vi "Formato de Archivo.vi"(8 "error in (no error)":errorcluster, 10 "Formato":enum16{"TXT", "TDMS"}(ring), 11 "Generador de Funciones in":refnum<class "Generador de Funciones.lvclass">) -> (0 "error out":errorcluster, 3 "Generador de Funciones out":refnum<class "Generador de Funciones.lvclass">)   [LabVIEW 2020, in "Generador de Funciones.lvlib" / "Generador de Funciones.lvclass"]
uses:
  Generador de Funciones.lvclass
  C:/Program Files (x86)/National Instruments/LabVIEW 2020/vi.lib/ActorFramework/Actor/Actor.lvclass
  Generador de Funciones.lvclass/Generador de Funciones.ctl
  Loggin/Loggin/Loggin.lvclass
  TDMS/TDMS/TDMS.lvclass
  <vilib>/ActorFramework/Message Enqueuer/Message Enqueuer.lvclass/Message Enqueuer.ctl
  <vilib>/ActorFramework/Message Enqueuer/Enqueue.vi
  <vilib>/ActorFramework/Stop Msg/Stop Msg.lvclass
  C:/Program Files (x86)/National Instruments/LabVIEW 2020/vi.lib/ActorFramework/Message/Message.lvclass
  <vilib>/ActorFramework/Message Priority Queue/Priority Enqueue.vi
  <vilib>/ActorFramework/Actor/Actor.lvclass
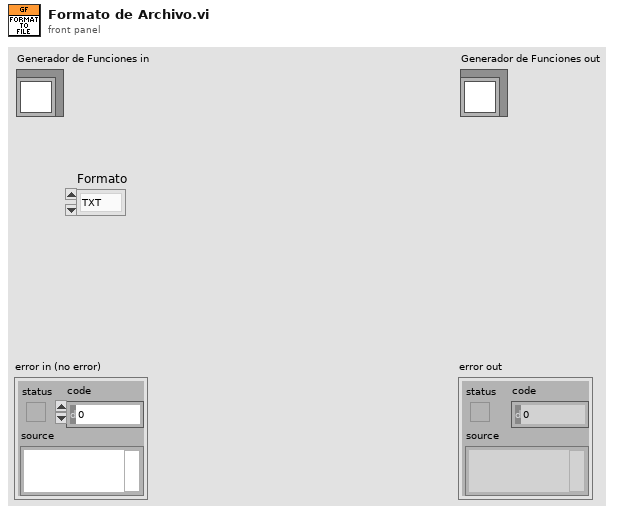
[diagram p1: front panel]
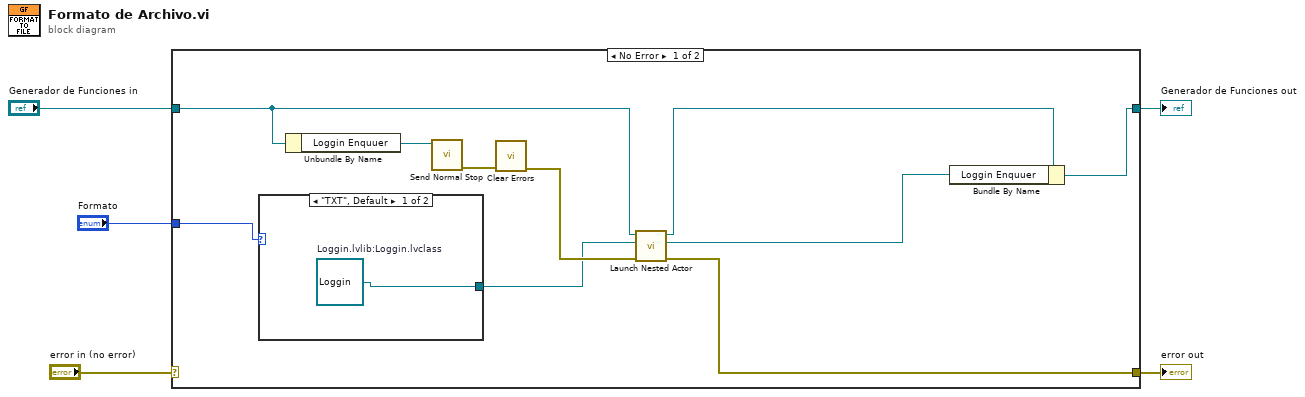
[diagram p0: block diagram]
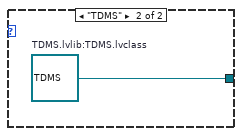
[diagram p2: hidden frame]
diagram:
  n1 = case shown="No Error" "error in (no error)" {
    selector: "error in (no error)" -> [_ w19]
    tunnel: [w10 w19] -> w4
    tunnel: [w8 w18] -> w2
    tunnel: "Generador de Funciones in" -> [w12 w18]
    tunnel: "Formato" -> [w13 _]
    frame No Error {
      n2 = case shown="\"TXT\", Default" w13 {
        tunnel: [w16 w17] -> w6
        frame "TXT", Default {
          w16 = refnum<class "Loggin.lvclass"> refnum  # Loggin.lvlib:Loggin.lvclass
        }
        frame "TDMS" {
          w17 = refnum<class "TDMS.lvclass"> refnum  # TDMS.lvlib:TDMS.lvclass
        }
      }
      n3 = Unbundle By Name(w12) -> ("Loggin Enquuer"=w15:refnum<class "Message Enqueuer.lvclass">)
      n4 = call <vilib>:"Send Normal Stop.vi"("Message Enqueuer"=w15) -> ("error out"=w14:errorcluster)  [unwired: 10 in]
      n5 = call <vilib>:"Clear Errors.vi"("error in (no error)"=w14) -> ("error out"=w11:errorcluster)  [unwired: 5 in, 1 out]
      n6 = call <vilib>:"Launch Nested Actor.vi"("error in (no error)"=w11, "Nested Actor"=w6, "Caller Actor in"=w12) -> ("error out"=w10:errorcluster, "Nested Actor's Enqueuer"=w7:refnum<class "Message Enqueuer.lvclass">, "Caller Actor out"=w9:refnum<class "Generador de Funciones.lvclass">)  [unwired: 6 in]
      n7 = Bundle By Name(cluster=w9, "Loggin Enquuer"=w7) -> (w8:refnum<class "Generador de Funciones.lvclass">)
    }
    frame Error {
    }
  }
  "error out" <- w4
  "Generador de Funciones out" <- w2
